vi "计算传感器值.vi"(10 "系数":sgl[](array[numeric]), 11 "电压值":sgl[](array[numeric])) -> (3 "传感器值":sgl[](array[numeric]))   [LabVIEW 2016]
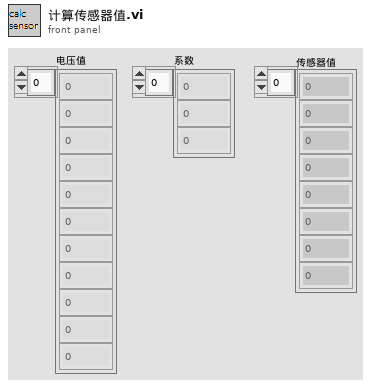
[diagram p1: front panel]
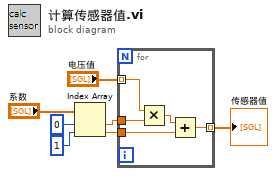
[diagram p0: block diagram]
diagram:
  n1 = Index Array(array="系数", index #1=0 ("索引"), index #2=1 ("索引")) -> (element #1=w3:sgl, element #2=w2:sgl)
  n2 = for {
    tunnel: "电压值" -> [w12] mode=indexing
    tunnel: w3 -> [w11]
    tunnel: w2 -> [w9]
    tunnel: [w8] -> w1 mode=indexing
    n3 = Multiply(x=w12, y=w11) -> (x*y=w10:sgl)
    n4 = Add(x=w10, y=w9) -> (x+y=w8:sgl)
  }
  "传感器值" <- w1
